vi "Send_amplitud.vi"(8 "error in (no error)":errorcluster, 10 "Amplitud":dbl, 11 "Signal_Gen in":refnum<class "Signal_Gen.lvclass">) -> (0 "error out":errorcluster, 3 "Signal_Gen out":refnum<class "Signal_Gen.lvclass">)   [LabVIEW 2019, in "Signal_Gen.lvlib" / "Signal_Gen.lvclass"]
uses:
  Signal_Gen.lvclass
  Signal_Gen.lvclass/Signal_Gen.ctl
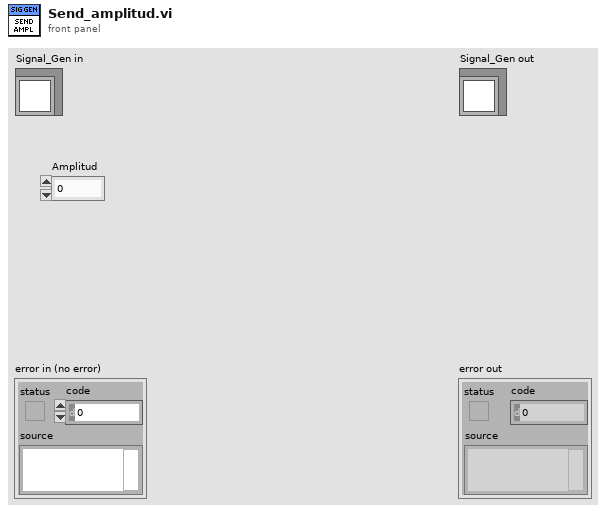
[diagram p1: front panel]
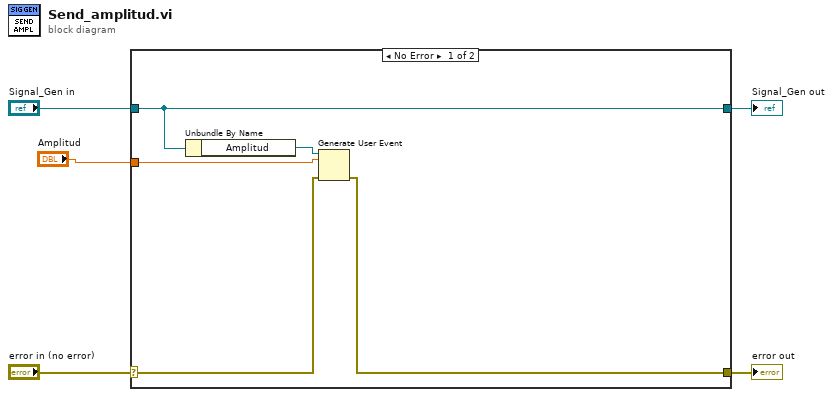
[diagram p0: block diagram]
diagram:
  n1 = case shown="No Error" "error in (no error)" {
    selector: "error in (no error)" -> [w7 w12]
    tunnel: [w6 w12] -> w4
    tunnel: [w10 w11] -> w2
    tunnel: "Signal_Gen in" -> [w10 w11]
    tunnel: "Amplitud" -> [w8 _]
    frame No Error {
      n2 = Unbundle By Name(w10) -> ("Amplitud"=w9:refnum<user-event>)
      n3 = Generate User Event(user event=w9, event data cluster=w8, error in=w7) -> (error out=w6:errorcluster)  [unwired: 1 in, 1 out]
    }
    frame Error {
    }
  }
  "error out" <- w4
  "Signal_Gen out" <- w2
